vi "Add2Stack&CheckThreshold.vi"(0 "Stack In":dbl[](array[numeric]), 1 "Stack Pointer  In":dbl, 2 "Stack Size":dbl, 3 "Angle":dbl, 4 "Threshold":dbl) -> (6 "Stack Out":dbl[](array[numeric]), 7 "Stack Pointer Out":dbl, 8 "Threshold Reached":bool)   [LabVIEW 2021]
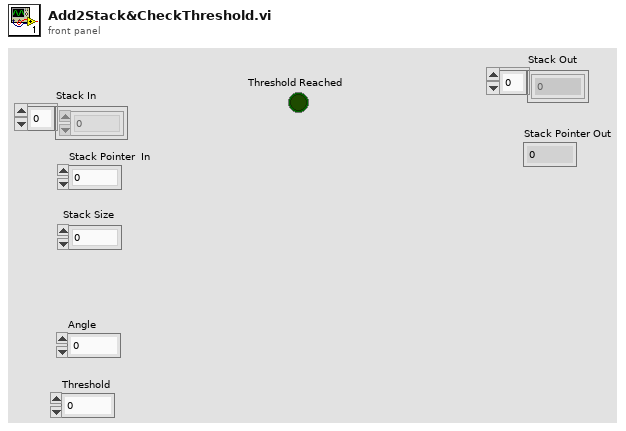
[diagram p1: front panel]
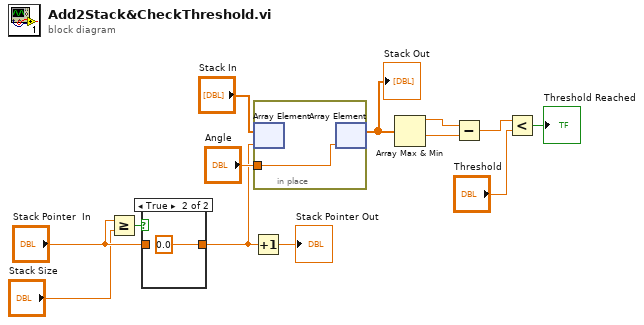
[diagram p0: block diagram]
diagram:
  n1 = Greater Or Equal?(x="Stack Pointer  In", y="Stack Size") -> (x >= y?=w3:bool)
  n2 = case shown="True" w3 {
    tunnel: [w14 0.0 ("Stack Pointer  In")] -> w6
    tunnel: "Stack Pointer  In" -> [w14 _]
    frame False {
    }
    frame True {
    }
  }
  n3 = Increment(x=w6) -> (x+1=→"Stack Pointer Out":dbl)
  n4 = in-place {
    in-place-border: "Angle" -> [w16]
    n5 = in-place-array #1("Stack In", w6) -> ()  [unwired: 1 out]
    n6 = in-place-array #1(w16) -> (w10:dbl[])  [unwired: 1 out]
  }
  "Stack Out" <- w10
  n7 = Array Max & Min(array=w10) -> (max value=w11:dbl, min value=w12:dbl)  [unwired: 2 out]
  n8 = Subtract(x=w11, y=w12) -> (x-y=w2:dbl)
  n9 = Less?(x=w2, y="Threshold") -> (x < y?=→"Threshold Reached":bool)
